vi "Loop_Timing.vi"(8 "error in":errorcluster) -> (0 "error out":errorcluster, 3 "Timing Block":T1 {"Actual Hz" format="%#_3g"; "Dt" format="%#_5g"; "Average Hz" format="%#_4g"})   [LabVIEW 2014]
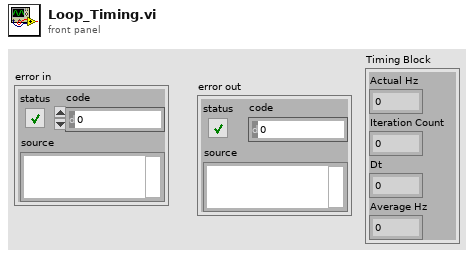
[diagram p1: front panel]
types:
  T1 = cluster{"Actual Hz":dbl, "Iteration Count":dbl, "Dt":dbl, "Average Hz":dbl}
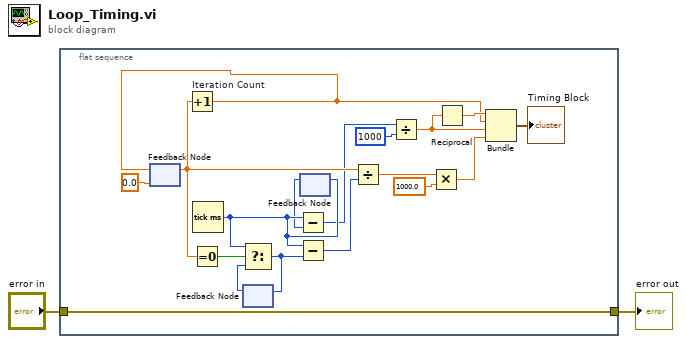
[diagram p0: block diagram]
diagram:
  n1 = flat-sequence {
    tunnel: "error in" -> [w4]
    tunnel: [w4] -> w1
    frame #0 {
      n2 = feedback #1(0.0) -> (w16:dbl)
      n3 = Increment "Iteration Count"(x=w16) -> (x+1=w3:dbl)
      n4 = feedback-in #1(w3) -> ()
      n5 = Equal To 0?(x=w16) -> (x = 0?=w17:bool)
      n6 = Tick Count (ms)() -> (millisecond timer value=w12:u32)
      n7 = feedback #2() -> (w18:u32)  [unwired: 1 in]
      n8 = Select(t=w12, s=w17, f=w18) -> (s? t:f=w19:u32)
      n9 = feedback-in #2(w19) -> ()
      n10 = Subtract(x=w12, y=w19) -> (x-y=w20:u32)
      n11 = feedback #3() -> (w11:u32)  [unwired: 1 in]
      n12 = Subtract(x=w12, y=w11) -> (x-y=w10:u32)
      n13 = feedback-in #3(w12) -> ()
      n14 = Divide(x=w16, y=w20) -> (x/y=w14:dbl)
      n15 = Divide(x=w10, y=u32 1000) -> (x/y=w6:dbl)
      n16 = Multiply(x=w14, y=1000.0) -> (x*y=w5:dbl)
      n17 = Reciprocal(x=w6) -> (1/x=w7:dbl)
      n18 = Bundle(w7, w3, w6, w5) -> (→"Timing Block":cluster{dbl, dbl, dbl, dbl})  [unwired: 1 in]
    }
  }
  "error out" <- w1
